vi "car3udpmsgtest01.vi"() -> ()   [LabVIEW 2020]
panel:
  in  "let_fail":bool
  out "parsed: sender port":u16=16100
  out "parsed: recv IP":string
  out "parsed: recv port":u16=16100
  out "error out":errorcluster
  out "parsed: data":string
  out "date/time string":string
  out "timestamp":dbl format="%.3f"
  out "parsed: msg_len":u16=1
  out "parsed: msg_type":u8=1
  out "parsed: sender IP":string
  in  "stop":bool
  in  "msg_type":u8
  in  "data (bytes string)":string="SB"
  in  "receiver_port":u16=16164
  in  "receiver_IPv4":string="192.168.232.64"
  in  "sender_port":u16=16101
  in  "sender_IPv4":string="192.168.232.1"
  out "message_bytes":string
  # "A test to make sure that compse.vi and parse.vi agree."
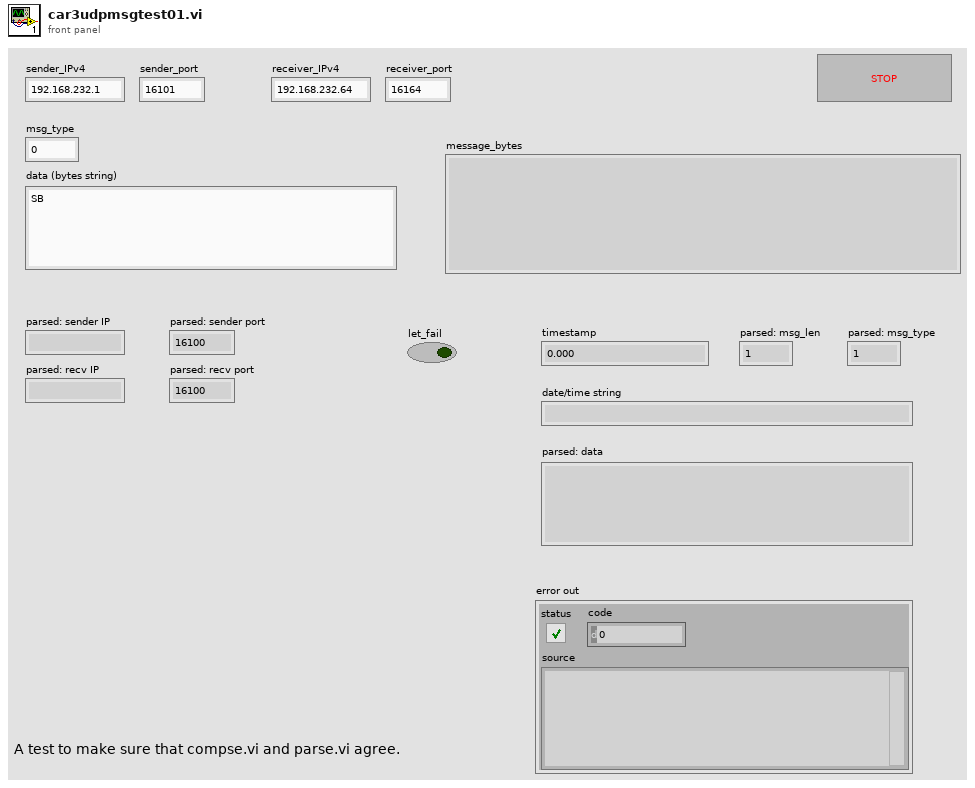
[diagram p1: front panel]
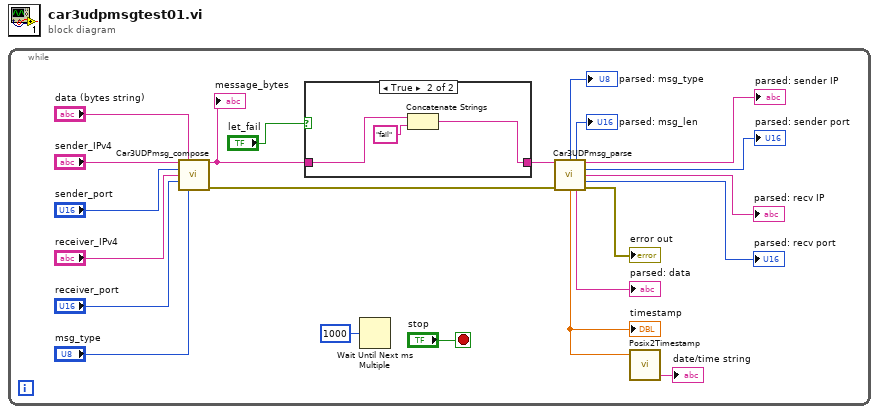
[diagram p0: block diagram]
diagram:
  n1 = while {
    stop <- "stop" stop-if-true
    n2 = call "Car3UDPmsg_compose.vi"("sender_IPv4"="sender_IPv4", "data (bytes string)"="data (bytes string)", "sender_port"="sender_port", "receiver_IPv4"="receiver_IPv4", "receiver_port"="receiver_port", "msg_type"="msg_type") -> ("message_bytes"=w2:string, "error out"=w14:errorcluster)  [unwired: 7 in, 1 out]
    "message_bytes" <- w2
    n3 = case shown="True" "let_fail" {
      tunnel: w2 -> [w23 w25]
      tunnel: [w23 w26] -> w1
      frame False {
      }
      frame True {
        n4 = Concatenate Strings(w25, "fail" ("string")) -> (w26:string)
      }
    }
    n5 = Wait Until Next ms Multiple(millisecond multiple=u32 1000) -> ()  [unwired: 1 out]
    n6 = call "Car3UDPmsg_parse.vi"("input (bytes string)"=w1, "error in (no error)"=w14) -> ("msg_type"=→"parsed: msg_type":u8, "msg_len"=→"parsed: msg_len":u16, "sender_IPv4"=→"parsed: sender IP":string, "sender_port"=→"parsed: sender port":u16, "receiver_IPv4"=→"parsed: recv IP":string, "receiver_port"=→"parsed: recv port":u16, "timestamp"=w10:dbl, "data (bytes string)"=→"parsed: data":string, "error out"=→"error out":errorcluster)  [unwired: 4 in, 1 out]
    "timestamp" <- w10
    n7 = call "Posix2Timestamp.vi"("POSIX"=w10) -> ("date/time string"=→"date/time string":string)  [unwired: 2 in, 2 out]
  }
